vi "CIC_5interpolate_5cycle.vi"(7 "reset":bool, 8 "valid in":bool, 11 "Data in":fxp<+/-,16,14>) -> (0 "valid out":bool, 3 "Data out":fxp<+/-,16,14>)   [LabVIEW 2018]
uses:
  <vilib>/rvi/IPIntegrationNode/IPINode_Typedef/niFpgaIPINodeSupportedFamilies.ctl
  <vilib>/rvi/IPIntegrationNode/IPINode_Utilities/niFpgaIPINodeSimCore.vi
  <vilib>/rvi/FXPMathLib/FxpMul/XNode/nifxpmath_Multiplier.xnode
  <vilib>/rvi/FXPMathLib/FxpInterpret/XNode/nifxpmath_Interpret.xnode
  <vilib>/rvi/XilinxIP/XIPIN_XNode/niFpgaXIPIN.xnode
  Xilinx/CIC_5interpolate_5cycle/CIC_5interpolate_5cycles/xsim.dir/CIC_5interpolate_5cycles_B599FC2E1D334E6F90A141D3DD2F38E2/xsimk_B599FC2E1D334E6F90A141D3DD2F38E2.dll
  <vilib>/rvi/IPIntegrationNode/IPINode_Xnode/niFpgaIPINode.xnode
  <vilib>/rvi/FXPMathLib/sim/FxpSim.dll
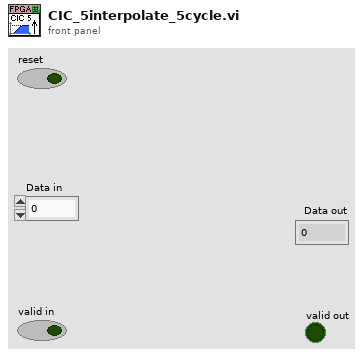
[diagram p1: front panel]
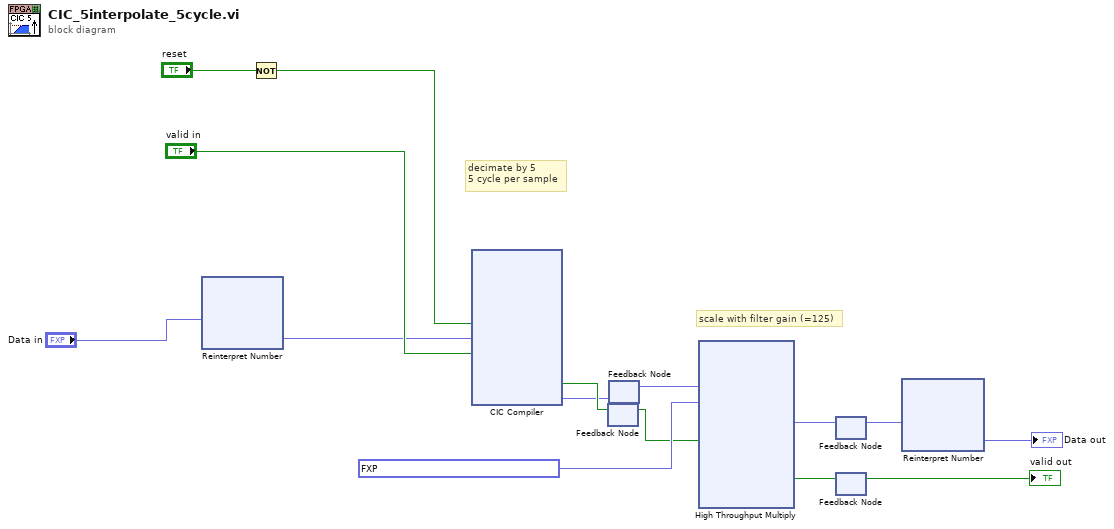
[diagram p0: block diagram]
diagram:
  # "decimate by 5\n5 cycle per sample"
  # "scale with filter gain (=125)"
  n1 = xnode "Reinterpret Number"("x"="Data in") -> ("y"=w3:fxp<+,16,16>)
  n2 = Not(x="reset") -> (.not. x?=w5:bool)
  n3 = xnode ("CIC Compiler")("aresetn"=w5, "s_axis_data_tdata"=w3, "s_axis_data_tvalid"="valid in") -> ("m_axis_data_tvalid"=w2:bool, "m_axis_data_tdata"=w1:fxp<+/-,24,24>)  [unwired: 1 in, 1 out]
  n4 = feedback #1() -> (w13:bool)  [unwired: 1 in]
  n5 = feedback-in #1(w2) -> ()
  n6 = feedback #2() -> (w12:fxp<+/-,24,24>)  [unwired: 1 in]
  n7 = feedback-in #2(w1) -> ()
  n8 = xnode ("High Throughput Multiply")("x"=w12, "y"=fxp<+/-,32,1> 0.007999999914318323, "input valid"=w13) -> ("x*y"=w9:fxp<+/-,16,16>, "output valid"=w8:bool)  [unwired: 1 in, 1 out]
  n9 = feedback #3() -> (w10:fxp<+/-,16,16>)  [unwired: 1 in]
  n10 = feedback-in #3(w9) -> ()
  n11 = feedback #4() -> (→"valid out":bool)  [unwired: 1 in]
  n12 = feedback-in #4(w8) -> ()
  n13 = xnode "Reinterpret Number"("x"=w10) -> ("y"=→"Data out":fxp<+/-,16,14>)
